vi "Get Items Visible.vi"(8 "error in (no error)":errorcluster, 10 "Return all? [T]":bool=TRUE, 11 "IContainer in":refnum<class "IContainer.lvclass">) -> (0 "error out":errorcluster, 2 "Visible":bool[](array[boolean]), 3 "IContainer out":refnum<class "IContainer.lvclass">, 4 "Items visible":bool[](array[boolean]))   [LabVIEW 2021, in "IContainer.lvclass"]
doc: "Copyright 2018, Wiebe Walstra, wiebe@carya.nl."
uses:
  IContainer.lvclass
  IContainer.lvclass/IContainer.ctl
  IObject.lvclass
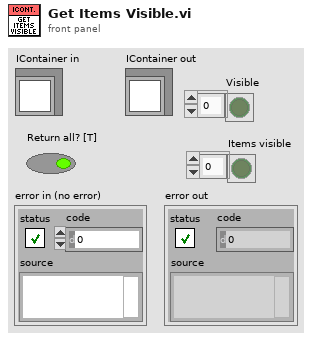
[diagram p1: front panel]
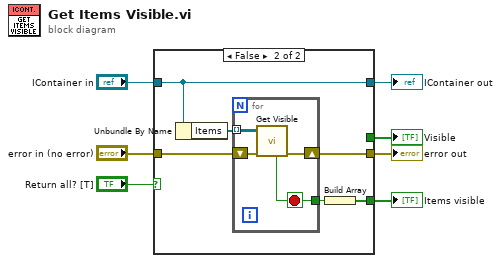
[diagram p0: block diagram]
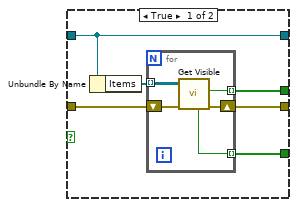
[diagram p2: hidden frame]
diagram:
  n1 = case shown="False" "Return all? [T]" {
    tunnel: [w13 w24] -> w7
    tunnel: "error in (no error)" -> [w12 w23]
    tunnel: [w11 _] -> w5
    tunnel: [w10 w19] -> w4
    tunnel: "IContainer in" -> [w8 w21]
    tunnel: [w8 w21] -> w2
    frame True {
      n2 = Unbundle By Name(w8) -> ("Items"=w9:refnum<class "IObject.lvclass">[])
      n3 = for {
        tunnel: w9 -> [w16] mode=indexing
        shift-right: [w17] -> w13
        shift-left: w12 -> [w18]
        tunnel: [w15] -> w11 mode=indexing
        tunnel: [w14] -> w10 mode=indexing
        n4 = call-dynamic "Get Visible.vi"("error in (no error)"=w18, "IObject in"=w16) -> ("error out"=w17:errorcluster, "Visible?"=w15:bool, "Item visible?"=w14:bool)  [unwired: 6 in, 1 out]
      }
    }
    frame False {
      n5 = Unbundle By Name(w21) -> ("Items"=w22:refnum<class "IObject.lvclass">[])
      n6 = for {
        tunnel: w22 -> [w26] mode=indexing
        shift-right: [w27] -> w24
        shift-left: w23 -> [w28]
        tunnel: [w25] -> w20
        stop <- w25 stop-if-true
        n7 = call-dynamic "Get Visible.vi"("error in (no error)"=w28, "IObject in"=w26) -> ("error out"=w27:errorcluster, "Item visible?"=w25:bool)  [unwired: 6 in, 2 out]
      }
      n8 = Build Array(w20) -> (w19:bool[])
    }
  }
  "error out" <- w7
  "IContainer out" <- w2
  "Visible" <- w5
  "Items visible" <- w4
